vi "Read Camera Temperature.vi"(8 "error in (no error)":errorcluster, 11 "Hamamatsu_C9100-13 in":refnum<class "Hamamatsu_C9100-13.lvclass">) -> (0 "error out":errorcluster, 2 "Camera Temperature":dbl, 3 "Hamamatsu_C9100-13 out":refnum<class "Hamamatsu_C9100-13.lvclass">)   [LabVIEW 2013, in "Hamamatsu_C9100-13.lvclass"]
uses:
  Hamamatsu_C9100-13.lvclass
  Hamamatsu_C9100-13.lvclass/Hamamatsu_C9100-13.ctl
  Globals.vi
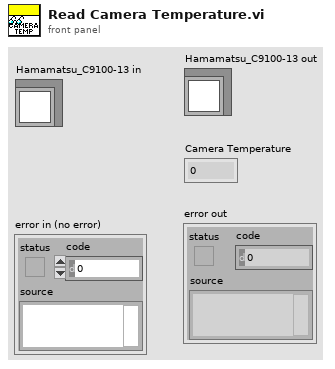
[diagram p1: front panel]
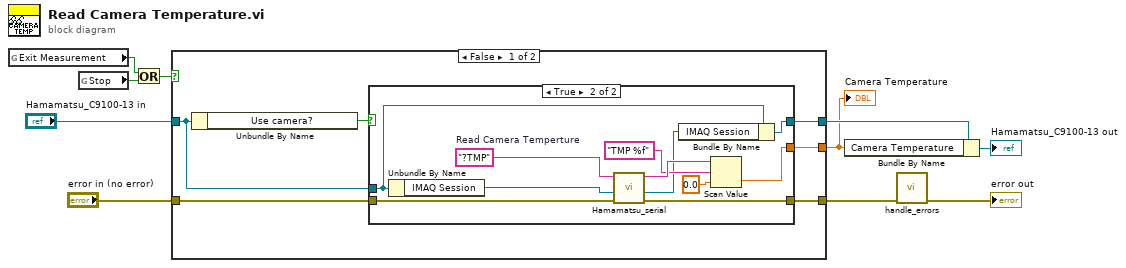
[diagram p0: block diagram]
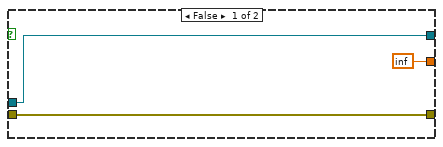
[diagram p2: hidden frame]
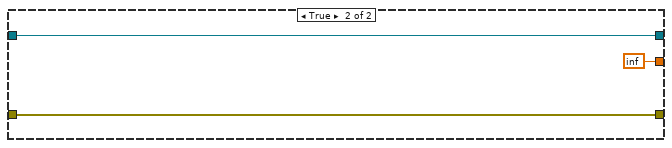
[diagram p3: hidden frame]
diagram:
  n1 = global read "Globals.vi" "Exit Measurement"() -> (w7:bool)
  n2 = global read "Globals.vi" "Stop"() -> (w6:bool)
  n3 = Or(x=w7, y=w6) -> (x .or. y?=w5:bool)
  n4 = case shown="False" w5 {
    tunnel: [w16 w31] -> w9
    tunnel: "Hamamatsu_C9100-13 in" -> [w11 w33]
    tunnel: [w14 inf] -> w1
    tunnel: [w15 w33] -> w3
    tunnel: "error in (no error)" -> [w12 w31]
    frame False {
      n5 = Unbundle By Name(w11) -> ("Use camera?"=w13:bool)
      n6 = case shown="True" w13 {
        tunnel: w12 -> [w19 w27]
        tunnel: [w19 w26] -> w16
        tunnel: [w18 w24] -> w15
        tunnel: [inf w20] -> w14
        tunnel: w11 -> [w18 w21]
        frame False {
        }
        frame True {
          w28 = "?TMP"  # Read Camera Temperture
          n7 = Unbundle By Name(w21) -> ("IMAQ Session"=w25:refnum<k11>)
          n8 = call "Hamamatsu_serial.vi"("error in"=w27, "IMAQ Session In"=w25, "Command to send"=w28) -> ("error out"=w26:errorcluster, "IMAQ Session Out"=w23:refnum<k11>, "Response from Camera"=w30:string)  [unwired: 6 in]
          n9 = Bundle By Name(cluster=w21, "IMAQ Session"=w23) -> (w24:refnum<class "Hamamatsu_C9100-13.lvclass">)
          n10 = Scan Value(string=w30, format string="TMP %f", default (0 dbl)=0.0 ("value (0)")) -> (value=w20:dbl)  [unwired: 1 out]
        }
      }
    }
    frame True {
    }
  }
  "Camera Temperature" <- w1
  n11 = Bundle By Name(cluster=w3, "Camera Temperature"=w1) -> (→"Hamamatsu_C9100-13 out":refnum<class "Hamamatsu_C9100-13.lvclass">)
  n12 = call "handle_errors.vi"("error in (no error)"=w9) -> ("error out"=→"error out":errorcluster)  [unwired: 14 in]
